vi "PerformScan_ESP.vi"(0 "ESP VISA":refnum<visa-resource-name>, 1 "Therapy/AVG ?":bool, 2 "Motion Settings":T1={"No Motion?"=FALSE, "Motion System"=enum."NI 735x", "Motion Bd ID"=1, "Motion Profile"="SMAC1", "# Axis"=1, "Reverse Z axis?"=TRUE, "SMAC Axis"=0, "scan pair"=enum."y-(x) scan", "RT fps"=6.0, "Steps per mm"=[1000, 1000, 1000, 1000], "Motor Parameters"={"velocity ct/s"=[10000.0, 10000.0, 10000.0, 50000.0], "accel ct/s^2"=[50000.0, 50000.0, 50000.0, 200000.0]}, "One Way Scan"=FALSE, "Reverse One Way Scan"=FALSE, "Global Position (mm)"=[], "Plane"=0, "Distance between\nscan lines (um)"=0.0, "Distance between\nscan planes (um)"=0.0, "number of scan planes"=1, "Total steps in line"=0, "Xtra plane\ndistance  (um)"=100, "Xtra planes "=1, "Add Axis"=FALSE, "overshoot cts"=200, "BKPT Shift"=0, "Scan Start Time (ms)"=0, "ESP VISA"="GPIB::1::INSTR", "3rd Axis"=1, "GL Ref Out"=refnum, "Galil Address"=""} {"3rd Axis" items=["x", "y", "z", "w"]; "Xtra planes" min=1; "Xtra plane\ndistance  (um)" min=0; "Distance between\nscan planes (um)" format="%.2f"; "Distance between\nscan lines (um)" format="%.2f"; "SMAC Axis" items=["None"=0, "Axis 1"=1, "Axis 2"=2, "Axis 3"=3, "Axis 4"=4, "Axis 5"=5, "Axis 6"=6, "Axis 7"=7, "Axis 8"=8, "Vector Space 1"=17, "Vector Space 2"=18, "Vector Space 3"=19, "Vector Space 4"=20]; "Motion Bd ID" min=1 max=32 step=1}, 5 "Line Axis":i32=1 min=1 max=4, 7 "Type of scan":T9, 9 "lines per scan plane":i32=128, 11 "Reverse ?":bool, 12 "Avg Num":i32=1, 13 "Digitizer Settings":T5={"Digitizer delay (us) "=0.0, "rf points per line"=2048, "lines per plane"=128, "Samp Rate (Hz)"=100000000.0, "Additional dig delay (us)"=0.0, "Voltage Scale"=0.4, "Pre-Looks"=0, "Offset delay (us)"=0.0, "bits A/D"=8, "Avg Num"=1, "DigTimeOut"=5.0, "Rel Dig Delay"=0.0, "Dig Ch"=0, "LeCroyCluster"={"LeCroy Channels"=[TRUE, FALSE, FALSE, FALSE], "LC read pt offset"=0.0, "Sweep Avg"=FALSE}, "Main Digitizer"=enum."NI Digitizer", "Dig Config"=enum."Single channel", "Digitizer ID Cluster"={"Acqiris/Alazar/SP ID"=[], "NI Instr Handles"=[], "LeCroy VISA"="", "GaGe Handle"={"Handle"=0, "Sample size"=0, "Resolution"=0, "Offset"=0, "Channels"=0, "Boards"=0}, "ATS Ref"="ATS9350", "Acqiris Address"=["PCI::INSTR0"], "ADQRef"=refnum, "adq_cu_ptr"=refnum}, "Trigger Settings"={"Trig Source"=1, "Trig Coupling"=0, "Trig Slope"=0, "Level (mV)"=1500.0}, "Bulk Acq"=FALSE, "Bulk Start Indexes"=[], "Data Ref RF"=refnum, "NI ID/Channel"=[], "Total Dig CH"=1, "Xtra Ann Trig delay (us)"=10.0, "Fix Z Delay?"=FALSE, "One Way Transmission?"=FALSE, "Data Ref Log"=refnum} {"Trigger Settings"."Trig Slope" items=["Positive", "Negative"]; "Trigger Settings"."Level (mV)" format="%.2f"; "Trigger Settings"."Trig Coupling" items=["DC 1 MOhm", "AC 1 MOhm", "DC 50 Ohm", "AC 50 Ohm"]; "Trigger Settings"."Trig Source" items=["Chan 1", "External"]; "Rel Dig Delay" format="%.2f"; "DigTimeOut" format="%.2f"; "Avg Num" min=1; "Offset delay (us)" format="%.2f"; "Additional dig delay (us)" format="%.2f"; "Digitizer delay (us)" format="%.2f"}, 14 "File Names":string[](array[string]), 15 "Offset":dbl format="%.2f") -> (4 "VISA resource name out":refnum<visa-resource-name>)   [LabVIEW 2022 SP3]
uses:
  -ScanSystem/Controls/ScanType2.ctl
  Digitizers/-DigitizerRoutines/DigitizerSettings.ctl
  Digitizers/-DigitizerRoutines/Digitizer.ctl
  Digitizers/-DigitizerRoutines/DigConfig.ctl
  Digitizers/-DigitizerRoutines/DigitizerID.ctl
  C:/Windows/System32/ADQAPI_dotNet_helper.dll
  NI_controller/-NI_MotionRoutines/MotionParameters.ctl
  NI_controller/-NI_MotionRoutines/MotionSys.ctl
  -MotionRoutines/ScanAxis.ctl
  -MotionRoutines/3rdAxis.ctl
  <instrlib>/Newport ESP301/Newport ESP301.lvlib
panel:
  # "allows movement down axis where pulse is sent out every time Step to Move has\nbeen moved. Small program is sent to MM2000 and executed. Motion is kind of slow."
  # "1-D and 2-D B scan settings"
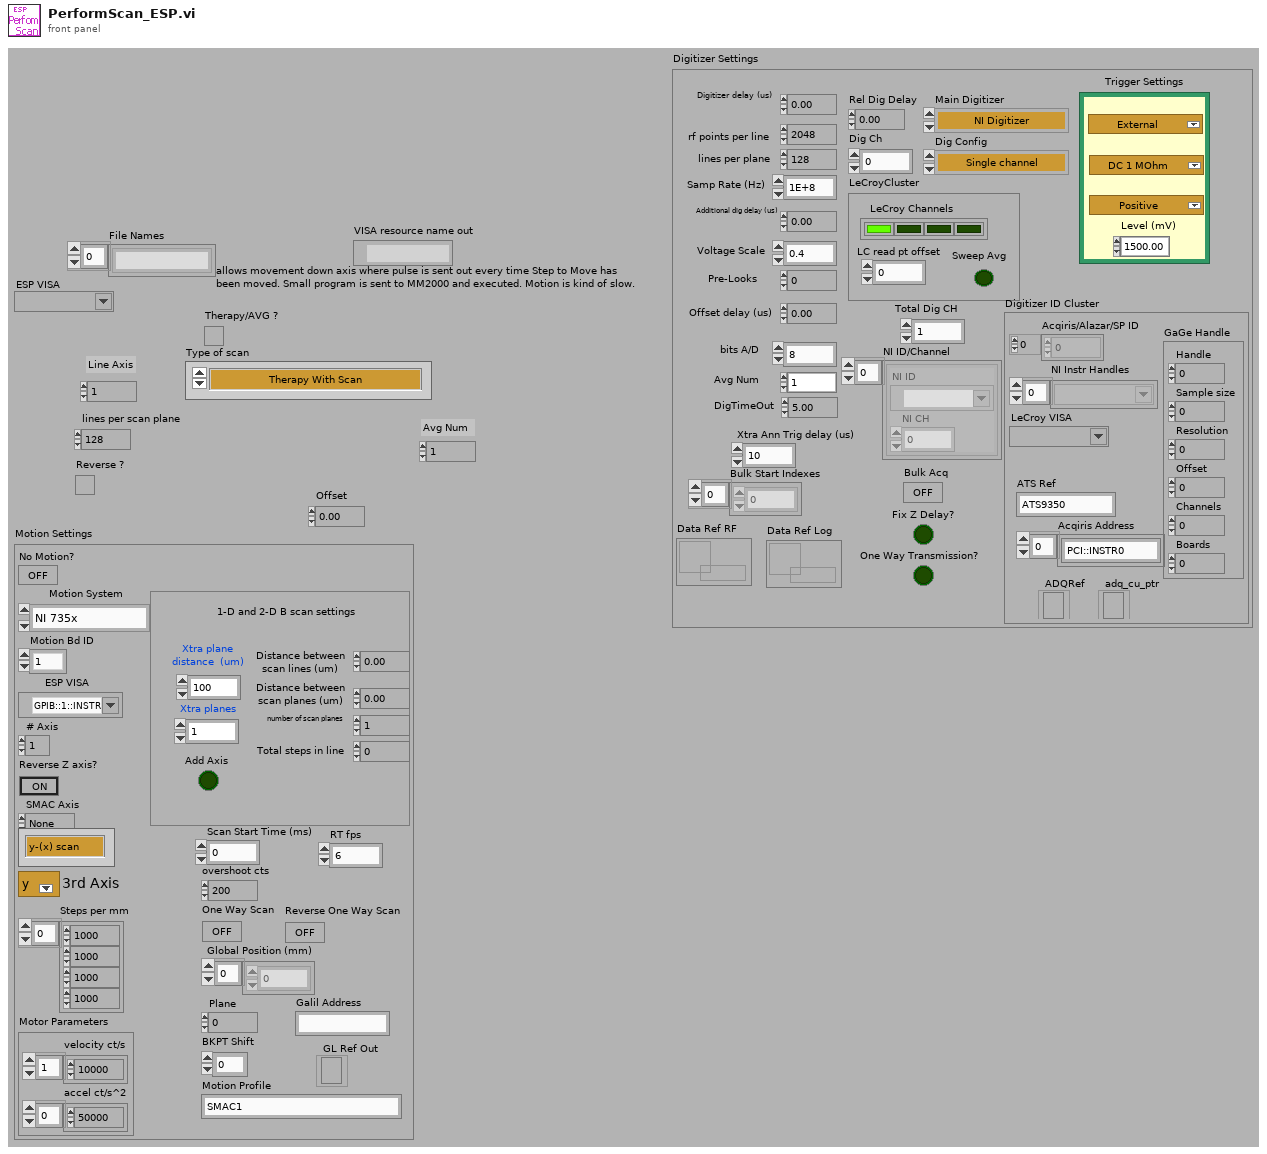
[diagram p1: front panel]
types:
  T1 = typedef "MotionParameters.ctl" = cluster{"No Motion?":bool, "Motion System":T2, "Motion Bd ID":u8, "Motion Profile":string, "# Axis":i8, "Reverse Z axis?":bool, "SMAC Axis":u16, "scan pair":T3, "RT fps":sgl, "Steps per mm":i32[], "Motor Parameters":cluster{"velocity ct/s":dbl[], "accel ct/s^2":dbl[]}, "One Way Scan":bool, "Reverse One Way Scan":bool, "Global Position (mm)":dbl[], "Plane":i32, "Distance between\nscan lines (um)":sgl, "Distance between\nscan planes (um)":sgl, "number of scan planes":i32, "Total steps in line":i32, "Xtra plane\ndistance  (um)":i32, "Xtra planes ":i32, "Add Axis":bool, "overshoot cts":i32, "BKPT Shift":i32, "Scan Start Time (ms)":u32, "ESP VISA":refnum<visa-resource-name>, "3rd Axis":T4, "GL Ref Out":refnum<k7>, "Galil Address":string}
  T2 = typedef "MotionSys.ctl" = enum16{"MM3000", "NI 735x", "Newport ESP", "No Motion Card", "Galil"}
  T3 = typedef "ScanAxis.ctl" = enum16{"y-(x) scan", "x-(y) scan", "z-(x) scan", "z-(y) scan", "y-(z) scan", "x-(z) scan", "w-(x) scan", "w-(y) scan", "w-(z) scan", "x-(w) scan", "y-(w) scan", "z-(w) scan"}
  T4 = typedef "3rdAxis.ctl" = u16
  T5 = typedef "DigitizerSettings.ctl" = cluster{"Digitizer delay (us) ":dbl, "rf points per line":i32, "lines per plane":i32, "Samp Rate (Hz)":dbl, "Additional dig delay (us)":dbl, "Voltage Scale":dbl, "Pre-Looks":i32, "Offset delay (us)":dbl, "bits A/D":i8, "Avg Num":i32, "DigTimeOut":sgl, "Rel Dig Delay":sgl, "Dig Ch":i32, "LeCroyCluster":cluster{"LeCroy Channels":bool[], "LC read pt offset":dbl, "Sweep Avg":bool}, "Main Digitizer":T6, "Dig Config":T7, "Digitizer ID Cluster":T8, "Trigger Settings":cluster{"Trig Source":u16, "Trig Coupling":u16, "Trig Slope":u16, "Level (mV)":dbl}, "Bulk Acq":bool, "Bulk Start Indexes":i32[], "Data Ref RF":refnum<data-value>, "NI ID/Channel":cluster{"NI ID":refnum<k15>, "NI CH":i32}[], "Total Dig CH":i32, "Xtra Ann Trig delay (us)":dbl, "Fix Z Delay?":bool, "One Way Transmission?":bool, "Data Ref Log":refnum<data-value>}
  T6 = typedef "Digitizer.ctl" = enum16{"Acqiris Digitizer", "NI Digitizer", "LeCroy", "GaGe", "AlazarTech", "No Digitizer", "Teledyne"}
  T7 = typedef "DigConfig.ctl" = enum16{"Single channel", "2 Chans w/ 2 Acqiris", "2 Chans w/ 1 Acqiris", "5-CH Pulser New", "5-CH pulser w/ ann array", "5-pass style ann array", "Empty"}
  T8 = typedef "DigitizerID.ctl" = cluster{"Acqiris/Alazar/SP ID":u32[], "NI Instr Handles":refnum<k15>[], "LeCroy VISA":refnum<visa-resource-name>, "GaGe Handle":cluster{"Handle":u32, "Sample size":u32, "Resolution":i32, "Offset":i32, "Channels":u32, "Boards":u32}, "ATS Ref":string, "Acqiris Address":string[], "ADQRef":refnum<k24>, "adq_cu_ptr":refnum<k24>}
  T9 = typedef "ScanType2.ctl" = enum16{"Therapy With Scan", "M scan", "M Scan With Therapy Burst", "1-D B Scan", "1-D B Scan With Therapy Burst", "2-D B Scan", "2-D B Scan With Therapy Burst", "Rotational Scan", "1-D B-Scan PRF", "2-D B-Scan PRF", "Real-Time Scan", "Contrast Agents", "1-D w/ Real-Time Set Up", "Dual Transducer", "Acoustic Microscopy", "Hydrophone Scanning"}
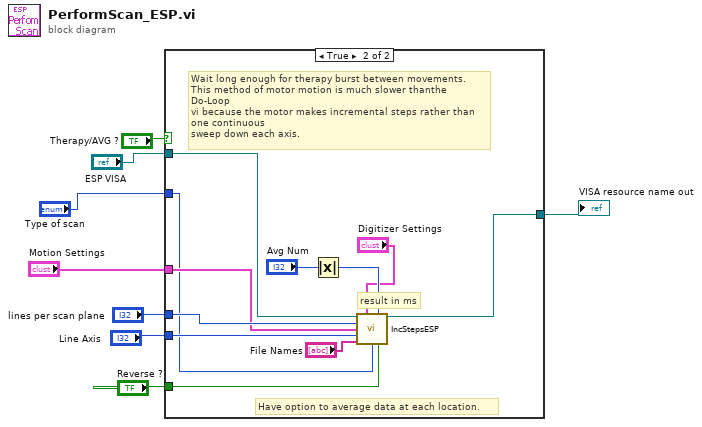
[diagram p0: block diagram]
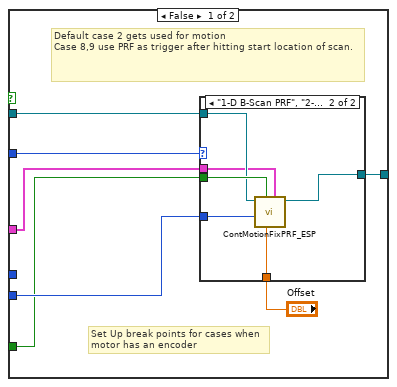
[diagram p2: hidden frame]
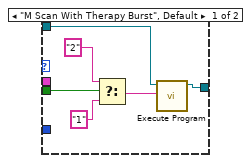
[diagram p3: hidden frame]
diagram:
  n1 = case shown="True" "Therapy/AVG ?" {
    tunnel: "Line Axis" -> [w15 w38]
    tunnel: "lines per scan plane" -> [_ w37]
    tunnel: "Reverse ?" -> [w14 w36]
    tunnel: "ESP VISA" -> [w12 w32]
    tunnel: [w11 w31] -> w4
    tunnel: "Motion Settings" -> [w10 w29]
    tunnel: "Type of scan" -> [w9 w28]
    frame False {
      # "Default case 2 gets used for motion\nCase 8,9 use PRF as trigger after hitting start location of scan."
      # "Set Up break points for cases when motor has an encoder"
      n2 = case shown="\"1-D B-Scan PRF\", \"2-D B-Scan PRF\"" w9 {
        tunnel: w15 -> [_ w24]
        tunnel: w14 -> [w21 w27]
        tunnel: "Offset" -> [_ w23]
        tunnel: w12 -> [w17 w26]
        tunnel: [w16 w25] -> w11
        tunnel: w10 -> [_ w22]
        frame "M Scan With Therapy Burst", Default {
          n3 = Select(t="2", s=w21, f="1") -> (s? t:f=w18:string)
          n4 = call <instrlib>:"Execute Program.vi"("Program Name"=w18, "VISA resource name"=w17) -> ("VISA resource name out"=w16:refnum<visa-resource-name>)  [unwired: 4 in, 1 out]
        }
        frame "1-D B-Scan PRF", "2-D B-Scan PRF" {
          n5 = call "ContMotionFixPRF_ESP.vi"("Motion Settings"=w22, "Offset"=w23, "Reverse ?"=w27, "Axis"=w24, "VISA resource name"=w26) -> ("VISA resource name out"=w25:refnum<visa-resource-name>)  [unwired: 5 in, 1 out]
        }
      }
    }
    frame True {
      # "Have option to average data at each location."
      # "Wait long enough for therapy burst between movements.\nThis method of motor motion is much slower thanthe Do-Loop\nvi because the motor makes incremental steps rather than one continuous\nsweep down each axis."
      # "result in ms"
      n6 = Absolute Value(x="Avg Num") -> (abs(x)=w33:i32)
      n7 = call "IncStepsESP.vi"("ESP VISA IN"=w32, "Digitizer Settings"="Digitizer Settings", "Avg Num"=w33, "number of scans"=w37, "Motion Settings"=w29, "Axis"=w38, "File Names"="File Names", "Type of scan"=w28, "Reverse ?"=w36) -> ("ESP VISA OUT"=w31:refnum<visa-resource-name>)  [unwired: 5 in, 1 out]
    }
  }
  "VISA resource name out" <- w4
